vi "Subvi timeout U32.vi"(8 "Timeout_tick":u32, 10 "Input":bool) -> (2 "Timeout":bool)   [LabVIEW 2017]
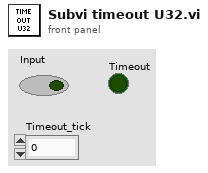
[diagram p1: front panel]
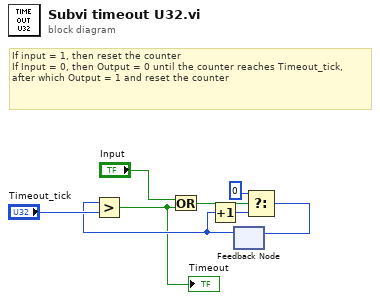
[diagram p0: block diagram]
diagram:
  # "If input = 1, then reset the counter\nIf Input = 0, then Output = 0 until the counter reaches Timeout_tick,\nafter which Output = 1 and reset the counter"
  n1 = feedback #1() -> (w4:u32)  [unwired: 1 in]
  n2 = Greater?(x=w4, y="Timeout_tick") -> (0:w3:bool)
  "Timeout" <- w3
  n3 = Or(x="Input", y=w3) -> (x .or. y?=w2:bool)
  n4 = Increment(x=w4) -> (x+1=w6:u32)
  n5 = Select(t=u32 0, s=w2, f=w6) -> (s? t:f=w5:u32)
  n6 = feedback-in #1(w5) -> ()
